vi "SummarizeFIFOTimes.vi"(1 "binning (s)":dbl format="%.2f", 2 "macro times (s)":u32[](array[numeric])) -> (0 "MCS":T1 {"binning (s)" format="%.2f"; "binning (s)" format="%.2f"})   [LabVIEW 2009]
uses:
  <vilib>/Analysis/NI_AALBase.lvlib
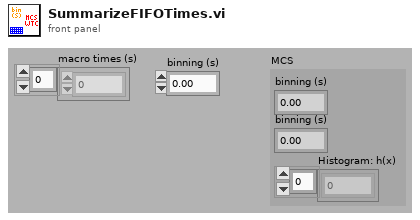
[diagram p1: front panel]
types:
  T1 = cluster{"binning (s)":dbl, "binning (s)":dbl, "Histogram: h(x)":i32[]}
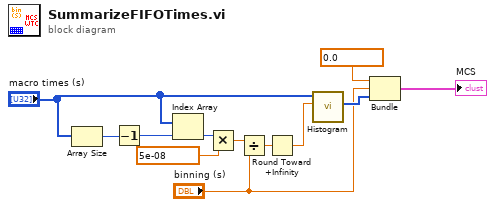
[diagram p0: block diagram]
diagram:
  n1 = Array Size(array="macro times (s)") -> (size(s)=w2:i32)
  n2 = Decrement(x=w2) -> (x-1=w3:i32)
  n3 = Index Array(array="macro times (s)", index=w3) -> (element=w4:u32)
  n4 = Multiply(x=w4, y=5e-08 ("binning (s)")) -> (x*y=w6:dbl)
  n5 = Divide(x=w6, y="binning (s)") -> (x/y=w7:dbl)
  n6 = Round Toward +Infinity(x=w7) -> (ceil(x): smallest int >= x=w8:dbl)
  n7 = call <vilib>:"Histogram.vi"("intervals"=w8, "X"="macro times (s)") -> ("Histogram: h(x)"=w10:i32[])  [unwired: 6 in, 3 out]
  n8 = Bundle("binning (s)"=0.0, "binning (s)"="binning (s)", "Histogram: h(x)"=w10) -> (→"MCS":T1)  [unwired: 1 in]
